vi "Export to csv.vi"(8 "error in (no error)":errorcluster, 11 "Table Data":string[][](array[string])) -> (0 "error out":errorcluster)   [LabVIEW 2017]
uses:
  <vilib>/Utility/file.llb/Write Delimited Spreadsheet (string).vi
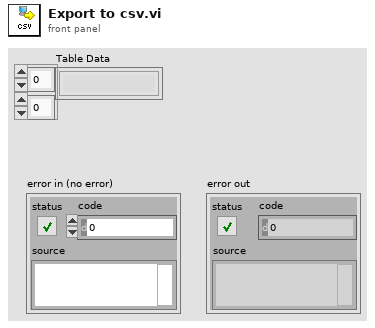
[diagram p1: front panel]
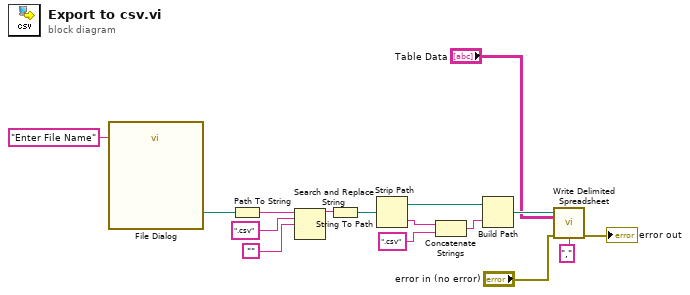
[diagram p0: block diagram]
diagram:
  n1 = call "File Dialog"("default name"="Enter File Name") -> ("selected path"=w13:path)  [unwired: 11 in, 3 out]
  n2 = Path To String(path=w13) -> (string=w12:string)
  n3 = Search and Replace String(input string=w12, search string=".csv", replace string="") -> (result string=w9:string)  [unwired: 5 in, 3 out]
  n4 = String To Path(string=w9) -> (path=w8:path)
  n5 = Strip Path(path=w8) -> (stripped path=w7:path, name=w15:string)
  n6 = Concatenate Strings(w15, ".csv" ("string")) -> (w6:string)
  n7 = Build Path(base path=w7, name or relative path=w6) -> (appended path=w5:path)
  n8 = call-poly <vilib>:"Write Delimited Spreadsheet.vi"("file path (dialog if empty)"=w5, "2D data"="Table Data", "error in (no error)"="error in (no error)", "delimiter (\\t)"="," ("delimiter (\\t)")) -> ("error out"=→"error out":errorcluster)  [unwired: 10 in, 1 out]
